vi "Edit Warning.vi"(7 "warning in":string) -> (3 "warning out":string)   [LabVIEW 2021, in "Converter.lvlib"]
uses:
  Converter.lvlib
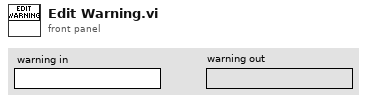
[diagram p1: front panel]
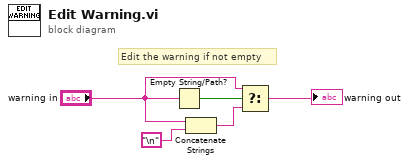
[diagram p0: block diagram]
diagram:
  # "Edit the warning if not empty"
  n1 = Empty String/Path?(string/path="warning in") -> (empty?=w3:bool)
  n2 = Concatenate Strings("warning in", "\n") -> (w5:string)
  n3 = Select(t="warning in", s=w3, f=w5) -> (s? t:f=→"warning out":string)
